vi "RSZVB Set Time Gate Sideband Suppression.vi"(8 "error in (no error)":errorcluster {"code" format="%.0x"}, 9 "Sideband Suppression (32.0 dB)":dbl=32.0 format="%^.3e", 10 "Channel (Trace) (1)":i32=1, 11 "VISA session":refnum<visa-resource-name>) -> (0 "error out":errorcluster {"code" format="%.0x"}, 3 "dup VISA session":refnum<visa-resource-name>)   [LabVIEW 2011]
doc: "This VI sets the sideband suppression for the Dolph-Chebyshev time gate. The command is only available if a Dolph-Chebyshev time gate is active.\n\nRemote-control command(s):\nCALCulate<Ch/Tr>:FILTer[:GATE]:TIME:DCHebyshev"
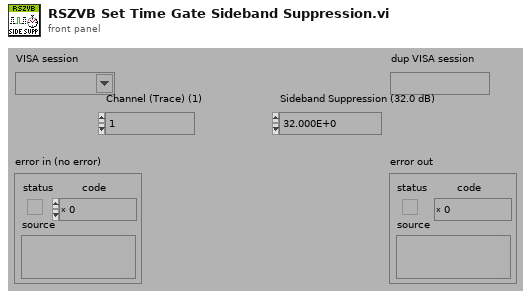
[diagram p1: front panel]
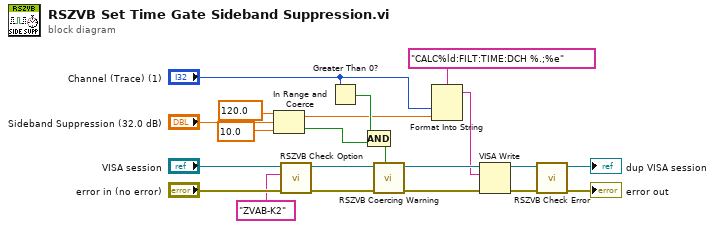
[diagram p0: block diagram]
diagram:
  n1 = In Range and Coerce(upper limit=120.0, x="Sideband Suppression (32.0 dB)", lower limit=10.0) -> (coerced(x)=w9:dbl, In Range?=w10:bool)
  n2 = call "RSZVB Check Option.vi"("error in (no error)"="error in (no error)", "Options"="ZVAB-K2", "VISA session"="VISA session") -> ("error out"=w8:errorcluster, "dup VISA session"=w13:refnum<visa-resource-name>)  [unwired: 7 in]
  n3 = Greater Than 0?(x="Channel (Trace) (1)") -> (x > 0?=w14:bool)
  n4 = Compound Arithmetic op=AND(w14, w10) -> (w16:bool)
  n5 = call "RSZVB Coercing Warning.vi"("In Range?"=w16, "error in (no error)"=w8, "VISA session"=w13) -> ("error out"=w19:errorcluster, "dup VISA session"=w20:refnum<visa-resource-name>)  [unwired: 7 in]
  n6 = Format Into String(format string="CALC%ld:FILT:TIME:DCH %.;%e", "Channel (Trace) (1)", w9) -> (resulting string=w15:string)  [unwired: 2 in, 1 out]
  n7 = VISA Write(VISA resource name=w20, write buffer=w15, error in (no error)=w19) -> (VISA resource name out=w17:refnum<visa-resource-name>, error out=w18:errorcluster)  [unwired: 1 out]
  n8 = call "RSZVB Check Error.vi"("error in (no error)"=w18, "VISA session"=w17) -> ("error out"=→"error out":errorcluster, "dup VISA session"=→"dup VISA session":refnum<visa-resource-name>)  [unwired: 8 in]
